vi "ApplyTableAppearance_benchmarking.vi"(6 "Defer Updates? (T)":bool=TRUE, 7 "Layout Ring Ref":refnum<vi>, 8 "error in (no error)":errorcluster, 9 "Mode Index":i32=2, 10 "Col Array in":refnum<class "Column.lvclass">[](array[class]), 11 "Table Ref in":refnum<vi>) -> (0 "error out":errorcluster, 3 "Table Ref out":refnum<vi>)   [LabVIEW 2013]
doc: "(Re)Initialize table appearance from column (appearance) array. A layout reference is required so that the existing layout view is preserved. The user can choose not to 'defer panel updates,' although the default is recommended to keep the program responsive.\n\nThis VI is read-only w.r.t. the column array."
uses:
  ColumnVIs/Column/Column.lvclass
  <vilib>/Utility/miscctls.llb/LVRowAndColumnTypeDef.ctl
  Globals/StdRowHeightGlobal.vi
panel:
  out "UnDefer (ms)":u32
  out "Layout (ms)":u32
  out "Rows + Mode (ms)":u32
  out "InitAppear (ms)":u32
  out "Reset Table (ms)":u32
  out "Defer (ms)":u32
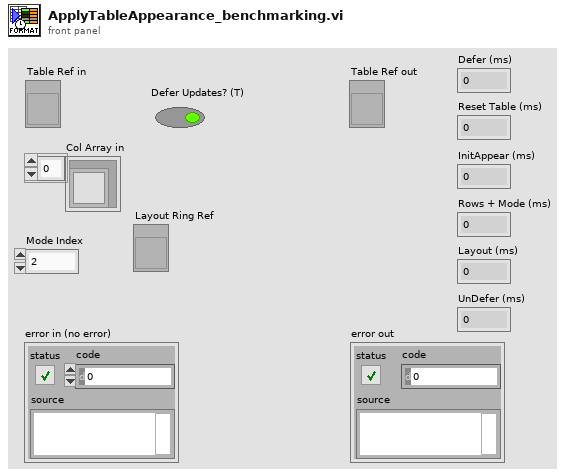
[diagram p1: front panel]
types:
  T1 = typedef "LVRowAndColumnTypeDef.ctl" = cluster{"Row":i32, "Column":i32}
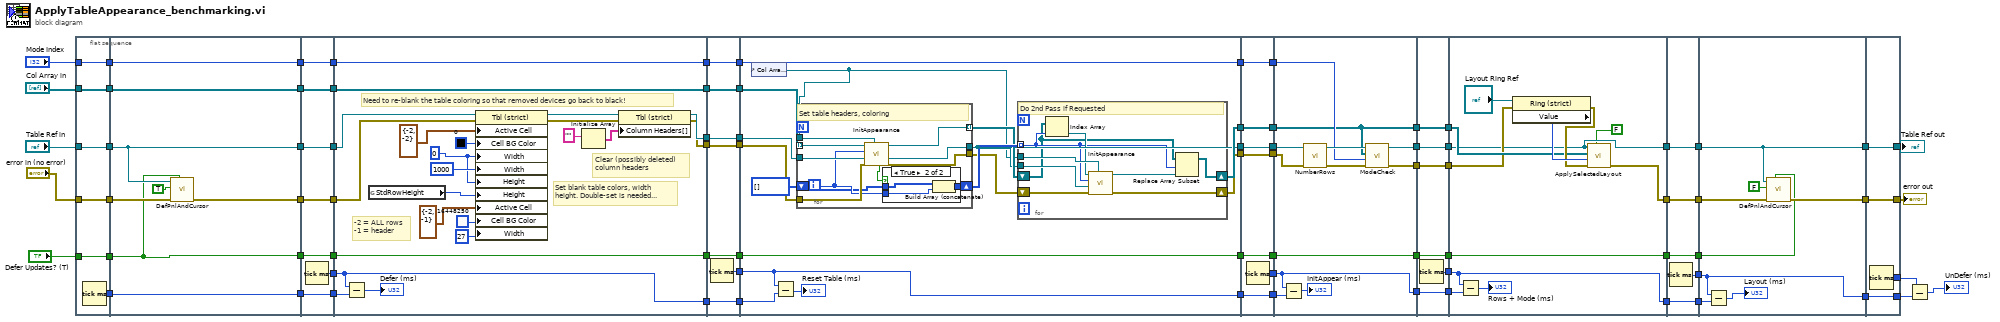
[diagram p0: block diagram]
diagram:
  n1 = flat-sequence {
    tunnel: "Mode Index" -> [w80]
    tunnel: "Col Array in" -> [w81]
    tunnel: "Table Ref in" -> [w82]
    tunnel: "Defer Updates? (T)" -> [w83]
    tunnel: "error in (no error)" -> [w84]
    tunnel: [w84] -> w70
    tunnel: [w83] -> w69
    tunnel: [w82] -> w68
    tunnel: [w81] -> w67
    tunnel: [w80] -> w66
    tunnel: [w79] -> w53
    tunnel: [w88] -> w65
    tunnel: [w87] -> w63
    tunnel: [w92] -> w61
    tunnel: [w91] -> w59
    tunnel: [w86] -> w57
    tunnel: w70 -> [w89]
    tunnel: w69 -> [w86]
    tunnel: w68 -> [w87]
    tunnel: w67 -> [w92]
    tunnel: w66 -> [w91]
    tunnel: [w90] -> w54
    tunnel: w53 -> [w90]
    tunnel: w65 -> [w99]
    tunnel: [w99] -> w64
    tunnel: w63 -> [w98]
    tunnel: [w98] -> w62
    tunnel: w61 -> [w97]
    tunnel: [w97] -> w60
    tunnel: w59 -> [w96]
    tunnel: [w96] -> w58
    tunnel: w57 -> [w95]
    tunnel: [w95] -> w56
    tunnel: [w94] -> w55
    tunnel: w54 -> [w94]
    tunnel: [w93] -> w52
    tunnel: w64 -> [w110]
    tunnel: w62 -> [w109]
    tunnel: w60 -> [w121]
    tunnel: w58 -> [w120]
    tunnel: [w111] -> w51
    tunnel: [w121] -> w49
    tunnel: [w120] -> w47
    tunnel: [w112] -> w45
    tunnel: w56 -> [w112]
    tunnel: [w108] -> w43
    tunnel: w55 -> [w106]
    tunnel: w52 -> [w105]
    tunnel: [w105] -> w40
    tunnel: w51 -> [w128]
    tunnel: [w128] -> w50
    tunnel: w49 -> [w127]
    tunnel: [w127] -> w48
    tunnel: w47 -> [w126]
    tunnel: [w126] -> w46
    tunnel: w45 -> [w125]
    tunnel: [w125] -> w44
    tunnel: w43 -> [w124]
    tunnel: [w124] -> w42
    tunnel: [w123] -> w41
    tunnel: w40 -> [w123]
    tunnel: [w122] -> w39
    tunnel: w50 -> [w141]
    tunnel: w48 -> [w143]
    tunnel: w46 -> [w144]
    tunnel: [w130] -> w38
    tunnel: [w144] -> w36
    tunnel: [w133] -> w34
    tunnel: [w142] -> w32
    tunnel: w44 -> [w142]
    tunnel: [w132] -> w30
    tunnel: w42 -> [w140]
    tunnel: w41 -> [w138]
    tunnel: w39 -> [w137]
    tunnel: [w137] -> w27
    tunnel: w38 -> [w175]
    tunnel: [w175] -> w37
    tunnel: w36 -> [w174]
    tunnel: [w174] -> w35
    tunnel: w34 -> [w173]
    tunnel: [w173] -> w33
    tunnel: w32 -> [w172]
    tunnel: [w172] -> w31
    tunnel: w30 -> [w171]
    tunnel: [w171] -> w29
    tunnel: [w170] -> w28
    tunnel: w27 -> [w170]
    tunnel: [w169] -> w26
    tunnel: w37 -> [w181]
    tunnel: w35 -> [w185]
    tunnel: [w180] -> w25
    tunnel: w33 -> [w184]
    tunnel: [w184] -> w23
    tunnel: w31 -> [w183]
    tunnel: [w183] -> w21
    tunnel: [w182] -> w19
    tunnel: w29 -> [w179]
    tunnel: w28 -> [w177]
    tunnel: w26 -> [w176]
    tunnel: [w176] -> w15
    tunnel: w25 -> [w193]
    tunnel: [w193] -> w24
    tunnel: w23 -> [w192]
    tunnel: [w192] -> w22
    tunnel: w21 -> [w191]
    tunnel: [w191] -> w20
    tunnel: w19 -> [w190]
    tunnel: [w190] -> w18
    tunnel: [w189] -> w17
    tunnel: [w188] -> w16
    tunnel: w15 -> [w188]
    tunnel: w24 -> [w198]
    tunnel: [w200] -> w14
    tunnel: [w198] -> w12
    tunnel: w22 -> [w202]
    tunnel: [w201] -> w10
    tunnel: w20 -> [w201]
    tunnel: w18 -> [w199]
    tunnel: w17 -> [w195]
    tunnel: w16 -> [w196]
    tunnel: [w195] -> w6
    tunnel: w14 -> [w210]
    tunnel: [w210] -> w13
    tunnel: w12 -> [w209]
    tunnel: [w209] -> w11
    tunnel: w10 -> [w208]
    tunnel: [w208] -> w9
    tunnel: [w207] -> w8
    tunnel: [w206] -> w7
    tunnel: w6 -> [w206]
    tunnel: w13 -> [w215]
    tunnel: w11 -> [w212]
    tunnel: w9 -> [w211]
    tunnel: w8 -> [w216]
    tunnel: w7 -> [w217]
    tunnel: [w214] -> w5
    tunnel: [w212] -> w4
    tunnel: [w216] -> w2
    tunnel: [w221] -> w73
    tunnel: [w222] -> w72
    tunnel: w5 -> [w222]
    tunnel: w4 -> [w221]
    tunnel: [w220] -> w3
    tunnel: w2 -> [w219]
    tunnel: [w219] -> w1
    frame #0 {
      n2 = Tick Count (ms)() -> (millisecond timer value=w79:u32)
    }
    frame #1 {
      n3 = call "DefPnlAndCursor.vi"("AllowDefPan? (T)"=w86, "error in (no error)"=w89, "DeferPanUpdts?"=TRUE, "Tbl Ctrl Refnum"=w87) -> ("error out"=w88:errorcluster)  [unwired: 7 in]
    }
    frame #2 {
      n4 = Tick Count (ms)() -> (millisecond timer value=w93:u32)
    }
    frame #3 {
      w101 = u32 0 ("Active Cell:Cell Size:Height")
      # "Clear (possibly deleted)\ncolumn headers"
      # "Need to re-blank the table coloring so that removed devices go back to black!"
      # "-2 = ALL rows\n-1 = header"
      # "Set blank table colors, width\nheight. Double-set is needed..."
      n5 = Subtract(x=w105, y=w106) -> (x-y=→"Defer (ms)":u32)
      n6 = global read "StdRowHeightGlobal.vi" "StdRowHeight"() -> (w102:u32)
      n7 = property class="Tbl (strict)"(reference=w109, error in=w110, "Active Cell"=T1 {"Row"=-2, "Column"=-2} ("RowAndCollumn"), "Cell BG Color"=u32 0, "Width"=w101, "Width"=u32 1000 ("Active Cell:Cell Size:Width"), "Height"=w101, "Height"=w102, "Active Cell"=T1 {"Row"=-2, "Column"=-1} ("RowAndCollumn"), "Cell BG Color"=u32 16448250, "Width"=u32 27 ("Active Cell:Cell Size:Width")) -> (reference out=w116:refnum<vi>, error out=w117:errorcluster)
      n8 = Initialize Array("") -> (w119:string[])  [unwired: 1 in]
      n9 = property class="Tbl (strict)"(reference=w116, error in=w117, "Column Headers[]"=w119) -> (reference out=w111:refnum<vi>, error out=w108:errorcluster)
    }
    frame #4 {
      n10 = Tick Count (ms)() -> (millisecond timer value=w122:u32)
    }
    frame #5 {
      n11 = control-ref of="Col Array in"() -> (w129:refnum<vi>)
      n12 = Subtract(x=w137, y=w138) -> (x-y=→"Reset Table (ms)":u32)
      n13 = for {
        tunnel: [w164] -> w131
        tunnel: [w163] -> w130
        tunnel: [w162] -> w134 mode=indexing
        tunnel: w143 -> [w158] mode=indexing
        tunnel: w141 -> [w161]
        tunnel: w140 -> [w160]
        tunnel: w129 -> [w159]
        shift-right: [w155] -> w135
        shift-left: i32[] [] -> [w154]
        i -> [w156]
        # "Set table headers, coloring"
        n14 = call-dynamic "InitAppearance.vi"("Col Array Ref in"=w159, "error in (no error)"=w160, "Table Ref in"=w161, "Col #"=w156, "Column in"=w158) -> ("error out"=w164:errorcluster, "Table Ref out"=w163:refnum<vi>, "Column out"=w162:refnum<class "Column.lvclass">, "Needs 2nd pass"=w157:bool)  [unwired: 3 in]
        n15 = case shown="True" w157 {
          tunnel: [w165 w168] -> w155
          tunnel: w156 -> [_ w167]
          tunnel: w154 -> [w165 w166]
          frame False {
          }
          frame True {
            n16 = Build Array (concatenate)(w166, w167) -> (w168:i32[])
          }
        }
      }
      n17 = for {
        tunnel: w129 -> [w150]
        tunnel: w130 -> [w153]
        shift-right: [w151] -> w132
        shift-left: w131 -> [w152]
        tunnel: w135 -> [w147] mode=indexing
        shift-right: [w146] -> w133
        shift-left: w134 -> [w145]
        # "Do 2nd Pass if Requested"
        n18 = Index Array(array=w145, index=w147) -> (element=w149:refnum<class "Column.lvclass">)
        n19 = call-dynamic "InitAppearance.vi"("Col Array Ref in"=w150, "error in (no error)"=w152, "Table Ref in"=w153, "Col #"=w147, "Column in"=w149) -> ("error out"=w151:errorcluster, "Column out"=w148:refnum<class "Column.lvclass">)  [unwired: 3 in, 2 out]
        n20 = Replace Array Subset(array=w145, new element=w148, index=w147) -> (w146:refnum<class "Column.lvclass">[])
      }
    }
    frame #6 {
      n21 = Tick Count (ms)() -> (millisecond timer value=w169:u32)
    }
    frame #7 {
      n22 = Subtract(x=w176, y=w177) -> (x-y=→"InitAppear (ms)":u32)
      n23 = call "NumberRows.vi"("error in (no error)"=w179, "Table Ref in"=w181) -> ("error out"=w186:errorcluster, "Table Ref out"=w187:refnum<vi>)  [unwired: 8 in]
      n24 = call "ModeCheck.vi"("error in (no error)"=w186, "mode col. index"=w185, "Col Array in"=w184, "Table Ref in"=w187) -> ("error out"=w182:errorcluster, "Table Ref out"=w180:refnum<vi>)  [unwired: 6 in]
    }
    frame #8 {
      n25 = Tick Count (ms)() -> (millisecond timer value=w189:u32)
    }
    frame #9 {
      n26 = Subtract(x=w195, y=w196) -> (x-y=→"Rows + Mode (ms)":u32)
      n27 = property class="Ring (strict)"(reference="Layout Ring Ref", error in=w199) -> (error out=w204:errorcluster, "Value"=w205:i32)  [unwired: 1 out]
      n28 = call "ApplySelectedLayout.vi"("Defer Updates? (T)"=FALSE, "error in (no error)"=w204, "Layout index"=w205, "Col array"=w202, "Tbl Refnum"=w198) -> ("error out"=w200:errorcluster)  [unwired: 6 in]
    }
    frame #10 {
      n29 = Tick Count (ms)() -> (millisecond timer value=w207:u32)
    }
    frame #11 {
      n30 = Subtract(x=w216, y=w217) -> (x-y=→"Layout (ms)":u32)
      n31 = call "DefPnlAndCursor.vi"("AllowDefPan? (T)"=w211, "error in (no error)"=w215, "DeferPanUpdts?"=FALSE, "Tbl Ctrl Refnum"=w212) -> ("error out"=w214:errorcluster)  [unwired: 7 in]
    }
    frame #12 {
      n32 = Tick Count (ms)() -> (millisecond timer value=w220:u32)
    }
  }
  n33 = Subtract(x=w3, y=w1) -> (x-y=→"UnDefer (ms)":u32)
  "error out" <- w72
  "Table Ref out" <- w73
